vi "ComplexFilter.vi"(0 "sampling_rate":dbl=1.0 format="%^.3e", 5 "vbw":dbl=300.0 caption="vbw_hz" format="%.2f", 7 "leading_first_point_samples":i32=100, 9 "bandwidths":dbl=300000.0 caption="bandwidth" format="%^.3e", 11 "min_selectivity":dbl=70.0 caption="min_selectivity1" format="%.2f", 12 "real_in":dbl[][](array[numeric]), 13 "imag_in":dbl[][](array[numeric])) -> (4 "FilteredData":dbl[][](array[numeric]))   [LabVIEW 2016]
uses:
  niRFUtil/Includes/niRFUtil INC Complex Waveform.ctl
  niRFUtil/Includes/niRFUtil INC Complex Array.ctl
  <vilib>/Analysis/baseanly.llb/Mean (DBL).vi
  <vilib>/Analysis/NI_AALBase.lvlib
  niRFUtil/niRFUtil.lvlib
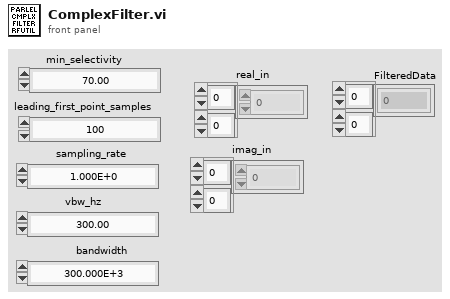
[diagram p1: front panel]
types:
  T1 = typedef "niRFUtil.lvlib/niRFUtil INC Complex Array.ctl" = csg[]
  T2 = typedef "niRFUtil.lvlib/niRFUtil INC Complex Waveform.ctl" = cluster{"x0":dbl, "dx":dbl, "y":T1}
  T3 = typedef "niRFUtil.lvlib/niRFUtil INC Real Waveform.ctl" = cluster{"x0":dbl, "dx":dbl, "y":T4}
  T4 = typedef "niRFUtil.lvlib/niRFUtil INC Real Array.ctl" = sgl[]
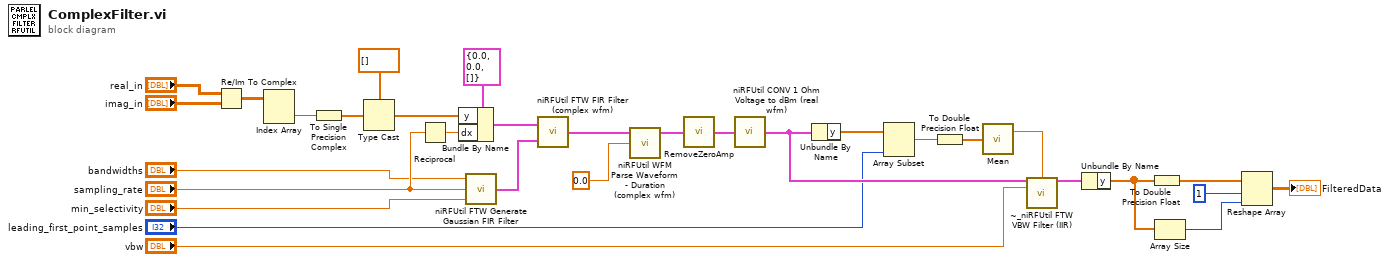
[diagram p0: block diagram]
diagram:
  n1 = Re/Im To Complex(1:"imag_in", 2:"real_in") -> (0:w8:cdb[][])
  n2 = Index Array(array=w8) -> (element=w7:cdb[])  [unwired: 2 in]
  n3 = To Single Precision Complex(1:w7) -> (0:w24:csg[])
  n4 = Type Cast(type=T1 [] ("y"), x=w24) -> (*(type *) &x=w27:T1)
  n5 = Reciprocal(x="sampling_rate") -> (1/x=w31:dbl)
  n6 = Bundle By Name(cluster=T2 {"x0"=0.0, "dx"=0.0, "y"=[]} ("Complex Waveform"), "y"=w27, "dx"=w31) -> (w30:T2)
  n7 = call "niRFUtil FTW Generate Gaussian FIR Filter.vi"("Minimum Selectivity (dB)"="min_selectivity", "Sampling Rate (Hz)"="sampling_rate", "Bandwidth (Hz)"="bandwidths") -> ("Filter"=w16:T3)
  n8 = call "niRFUtil FTW FIR Filter (complex wfm).vi"("Filter"=w16, "Waveform In"=w30) -> ("Waveform Out"=w15:T2)
  n9 = call "niRFUtil WFM Parse Waveform - Duration (complex wfm).vi"("Start (-Inf)"=0.0 ("Start"), "Waveform In"=w15) -> ("Waveform Out"=w13:T2)  [unwired: 3 in]
  n10 = call "RemoveZeroAmp.vi"("Complex Waveform In"=w13) -> ("Real Waveform out"=w12:T3)  [unwired: 14 in]
  n11 = call "niRFUtil CONV 1 Ohm Voltage to dBm (real wfm).vi"("Real Waveform (V)"=w12) -> ("Real Waveform (dBm)"=w11:T3)  [unwired: 14 in]
  n12 = Unbundle By Name(w11) -> ("y"=w3:T4)
  n13 = Array Subset(array=w3, length="leading_first_point_samples") -> (w1:T4)  [unwired: 1 in]
  n14 = To Double Precision Float(number=w1) -> (double precision float=w17:dbl[])
  n15 = call-poly <vilib>:"Mean.vi"("X"=w17) -> ("mean"=w18:dbl)  [unwired: 1 out]
  n16 = call "~_niRFUtil FTW VBW Filter (IIR).vi"("Waveform In"=w11, "Initial Condition"=w18, "VBW (Hz)"="vbw") -> ("Waveform Out"=w19:T3)  [unwired: 12 in]
  n17 = Unbundle By Name(w19) -> ("y"=w6:T4)
  n18 = To Double Precision Float(number=w6) -> (double precision float=w9:dbl[])
  n19 = Array Size(array=w6) -> (size(s)=w5:i32)
  n20 = Reshape Array(w9, 1 ("dimension size"), w5) -> (→"FilteredData":dbl[][])
